vi "CTO.vi"(0 "System no.":i32=1 min=1 max=4 step=1, 2 "TriggerOut to set":string[](array[string]), 4 "No.of digits":i16=4, 5 "error in":errorcluster, 6 "CTO parameter ID":i32[](array[numeric]), 10 "Parameter value":string[](array[string])) -> (14 "Controller error":bool, 19 "error out":errorcluster)   [LabVIEW 2020]
doc: "This VI configures the trigger output conditions for the given trigger output line, waits 100 ms and queries ERR?. The trigger output will always be periodically. The trigger output only becomes active when enabled with TRO. Note: Do not use DIO when an axis was configured with CTO. See user manual or GCS DLL manual for available parameter numbers and values. No. of digits is the number of digits after the decimal point in the numeric parameter value(s) that will be sent. Controller error is TRUE if selected system reports error code not equal to 0. \n\nC-413: TriggerOut to set can be 1 to 5.\n\nC-702: TriggerOut to set can be 1 to 8. DIO uses A-H to designate the same lines CTO calls 1-8.\n\nC-843: TriggerOut to set can be 1 to 4 (4-axis card) or 2 (2-axis card).\n\nC-866: TriggerOut to set can be 1.\n\nC-867, C-877: Check controller user manual for available output trigger numbers. \n\nC-884, E-871, E-873, E-874: Check C-884 user manual for available output trigger numbers. \n\nE-517, E-518: TriggerOut to set can be 1 to 3.The trigger output is immediately active when the condition given by the CTO configuration is fulfilled (there is no TRO command). If the CTO Parameter ID is \"Trigger Mode\" and the Parameter value is \"Generator Trigger\", then the trigger points in the waveform must be set with TWS and/or with WGO.\nThe current trigger output configuration is saved with the WPA command, in addition to the current parameter values and other settings. \nThe width of a trigger pulse is 30 µs by default, except with the MinMaxThreshold trigger mode where the pulse width depends on the threshold settings. You can change the default pulse width using the Pulse Width parameter, ID 0x0E000900. Possible values are in the range of 10 to 150 µs.\nThe assignment of the trigger lines to the axes of the controller is fixed (DIO_O1 belongs to the first axis (A by default), DIO_O2 to the second axis (B by default) and DIO_O3 to the third axis (C by default).\n\nE-709: TriggerOut to set can be 1 to 2. The trigger output is immediately active when the condition given by the CTO configuration is fulfilled (there is no TRO command). If the CTO Parameter ID is \"Trigger Mode\" and the Parameter value is \"Generator Trigger\", then the trigger points in the waveform must be set with TWS. \n\nE-712: TriggerOut to set can be 1 to 7. The trigger output is immediately active when the condition given by the CTO configuration is fulfilled (there is no TRO command). If the CTO Parameter ID is \"Trigger Mode\" and the Parameter value is \"Generator Trigger\", then the trigger points in the waveform must be set with TWS. By default, axis 1 is connected to TriggerOut line 1, axis 2 to line 2, axis 3 to line 3, ..., axis n to line n. If the number of TriggerOut lines exceeds the number of axes, the \"surplus\" lines are all connected to the last axis.\n\nE-725: TriggerOut to set can be 1 to 7. The trigger output is immediately active when the condition given by the CTO configuration is fulfilled (there is no TRO command). If the CTO Parameter ID is \"Trigger Mode\" and the Parameter value is \"Generator Trigger\", then the trigger points in the waveform must be set with TWS. By default, axis 1 is connected to TriggerOut line 1, axis 2 to line 2, axis 3 to line 3, ..., axis n to line n. If the number of TriggerOut lines exceeds the number of axes, the \"surplus\" lines are all connected to the last axis.\n\nE-727: TriggerOut to set can be 1 to 3.The trigger output is immediately active when the condition given by the CTO configuration is fulfilled (there is no TRO command). If the CTO Parameter ID is \"Trigger Mode\" and the Parameter value is \"Generator Trigger\", then the trigger points in the waveform must be set with TWS. By default, axis 1 is connected to TriggerOut line 1, axis 2 to line 2, axis 3 to line 3. If the number of TriggerOut lines exceeds the number of axes, the \"surplus\" lines are all connected to the last axis.\n\nE-753: TriggerOut to set can be 1. The trigger output is immediately active when the condition given by the CTO configuration is fulfilled (there is no TRO command). If the CTO Parameter ID is \"Trigger Mode\" and the Parameter value is \"Generator Trigger\", then the trigger points in the waveform must be set with TWS. \n\nE-754: TriggerOut to set can be 1. The trigger output is immediately active when the condition given by the CTO configuration is fulfilled (there is no TRO command). If the CTO Parameter ID is \"Trigger Mode\" and the Parameter value is \"Generator Trigger\", then the trigger points in the waveform must be set with TWS. \n\nMercury: TriggerOut to set can be 1 to N (N: number of connected axes, if supported by corresponding Mercury firmware).\n\nMercury_GCS: Check Mercury user manual for available output trigger numbers."
panel:
  # "This vi Configures the Trigger Output conditions for the given trigger output line, waits\n100 ms and queries ERR?. The trigger output will always be periodically. The trigger \noutput only becomes active when enabled with TRO. Note: Do not use DIO when an axis \nwas configured with CTO."
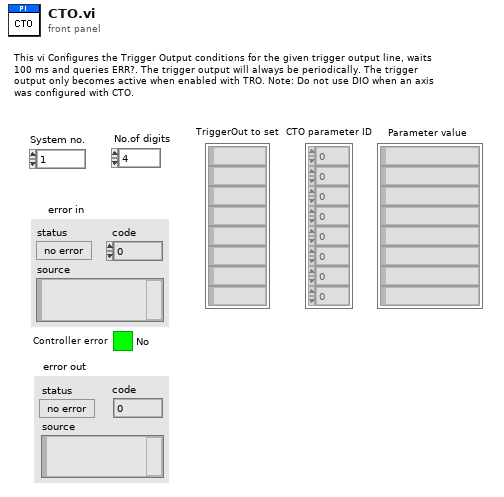
[diagram p1: front panel]
types:
  T1 = enum16{"Disable error check", "Force error check", "Use global settings"}
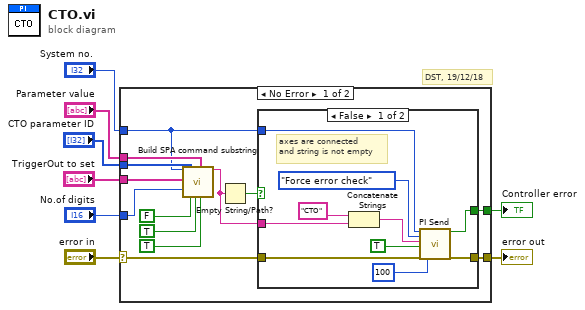
[diagram p0: block diagram]
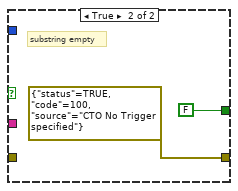
[diagram p2: hidden frame]
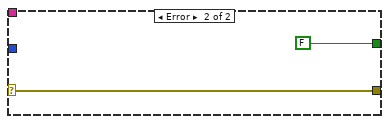
[diagram p3: hidden frame]
diagram:
  # "DST, 19/12/18"
  n1 = case shown="No Error" "error in" {
    selector: "error in" -> [w9 w34]
    tunnel: [w21 w34] -> w8
    tunnel: "No.of digits" -> [w20 _]
    tunnel: "System no." -> [w16 _]
    tunnel: "TriggerOut to set" -> [w19 _]
    tunnel: "CTO parameter ID" -> [w18 _]
    tunnel: "Parameter value" -> [w17 _]
    tunnel: [w12 FALSE ("Controller error")] -> w2
    frame No Error {
      n2 = call "Build SPA command substring.vi"("System no."=w16, "Axes to set"=w19, "No. of digits"=w20, "Parameter number"=w18, "Parameter no. format \n(Decimal: FALSE)"=FALSE ("Parameter no. format \n(Decimal: FALSE)"), "Parameter format \n(Num.: FALSE)"=TRUE ("Parameter format \n(Num.: FALSE)"), "Parameter strings"=w17, "With space?"=TRUE) -> ("SPA command substring"=w11:string)  [unwired: 2 in, 9 out]
      n3 = Empty String/Path?(string/path=w11) -> (empty?=w10:bool)
      n4 = case shown="False" w10 {
        tunnel: w11 -> [w30 _]
        tunnel: [w24 errorcluster {"status"=TRUE, "code"=100, "source"="CTO No Trigger specified"} ("error out")] -> w21
        tunnel: w9 -> [w27 _]
        tunnel: w16 -> [w26 _]
        tunnel: [w23 FALSE ("Controller error")] -> w12
        frame False {
          # "axes are connected \nand string is not empty"
          n5 = Concatenate Strings("CTO", w30) -> (w28:string)
          n6 = call "PI Send.vi"("System no."=w26, "Error check settings"=T1."Force error check", "String to send"=w28, "Attach termination char.?"=TRUE ("Attach Linefeed?"), "error in"=w27, "Delay before error check (ms)"=u32 100 ("milliseconds to wait")) -> ("Controller error"=w23:bool, "error out"=w24:errorcluster)  [unwired: 12 out]
        }
        frame True {
          # "substring empty"
        }
      }
    }
    frame Error {
    }
  }
  "error out" <- w8
  "Controller error" <- w2
